vi "Sensor List2String.vi"(8 "error in (no error)":errorcluster, 11 "Sensor List Class in":refnum<class "Sensor List Class.lvclass">) -> (0 "error out":errorcluster, 2 "Strings":string[][](array[string]), 3 "Sensor List Class out":refnum<class "Sensor List Class.lvclass">)   [LabVIEW 2013, in "Sensor List Class.lvclass"]
uses:
  Sensor List Class.lvclass
  W:/NSEL OM/lib/Data Access Objects/Sensors/Sensor DAO Class.lvclass
  Sensor List Class.lvclass/Sensor List Class.ctl
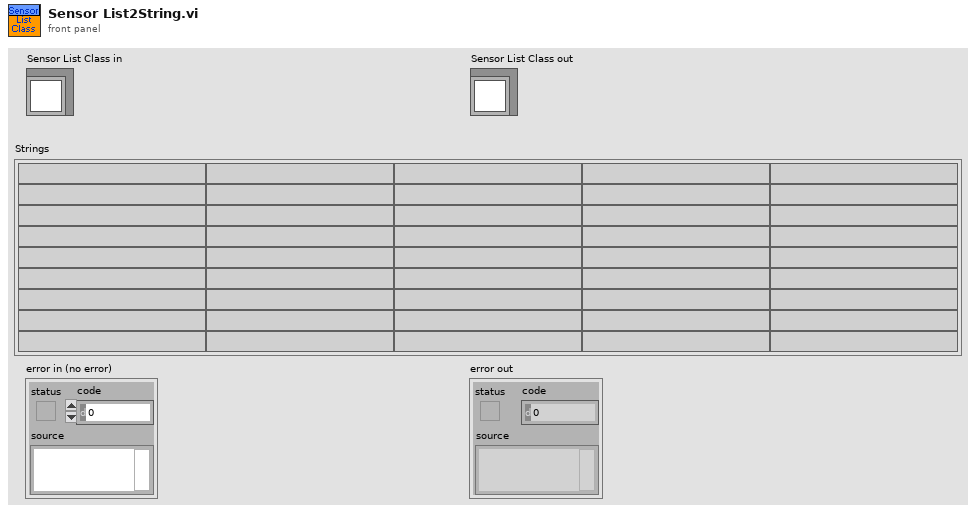
[diagram p1: front panel]
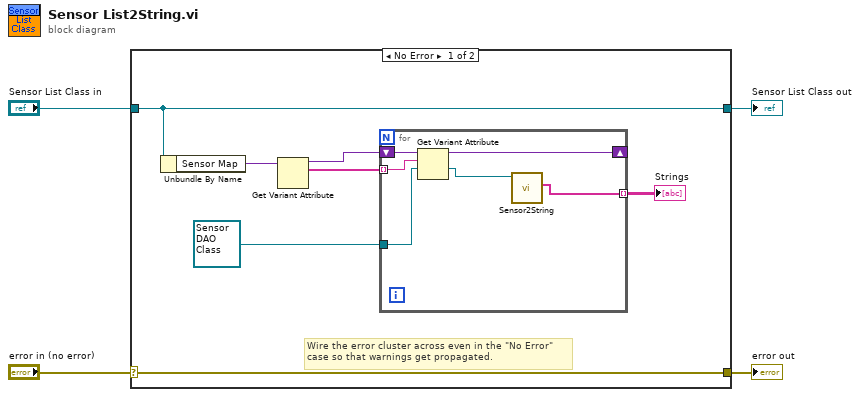
[diagram p0: block diagram]
diagram:
  n1 = case shown="No Error" "error in (no error)" {
    selector: "error in (no error)" -> [w11 w19]
    tunnel: [w11 w19] -> w3
    tunnel: [w10 w18] -> w1
    tunnel: "Sensor List Class in" -> [w10 w18]
    frame No Error {
      # "Wire the error cluster across even in the \"No Error\"\ncase so that warnings get propagated."
      n2 = Unbundle By Name(w10) -> ("Sensor Map"=w9:variant)
      n3 = Get Variant Attribute(Variant=w9) -> (duplicate Variant=w7:variant, names=w8:string[])  [unwired: 3 in, 2 out]
      n4 = for {
        tunnel: w8 -> [w17] mode=indexing
        shift-right: [w15] -> _
        shift-left: w7 -> [w16]
        tunnel: refnum<class "Sensor DAO Class.lvclass"> refnum ("Sensor DAO Class.lvclass") -> [w14]
        tunnel: [w12] -> w5 mode=indexing
        n5 = Get Variant Attribute(Variant=w16, name=w17, default value (empty Variant)=w14) -> (duplicate Variant=w15:variant, value=w13:refnum<class "Sensor DAO Class.lvclass">)  [unwired: 1 in, 2 out]
        n6 = call "Sensor2String.vi"("Sensor DAO Class in"=w13) -> ("Strings"=w12:string[])  [unwired: 8 in, 2 out]
      }
      "Strings" <- w5
    }
    frame Error {
    }
  }
  "error out" <- w3
  "Sensor List Class out" <- w1
